vi "Creat Select cmd.vi"(0 "Col":string, 1 "Code":string, 3 "Condtion":string) -> (2 "连接的字符串":string, 4 "Str":string)   [LabVIEW 2014]
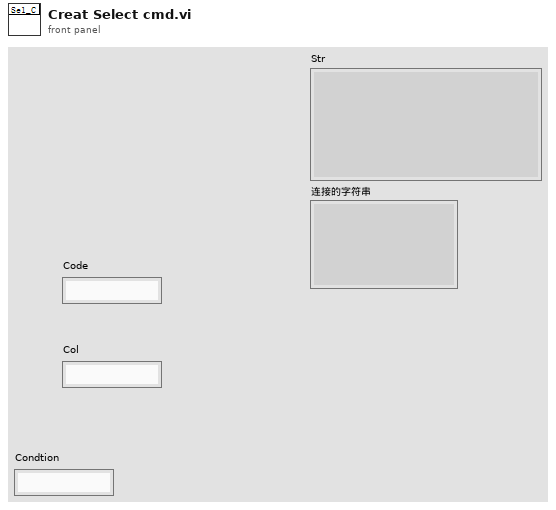
[diagram p1: front panel]
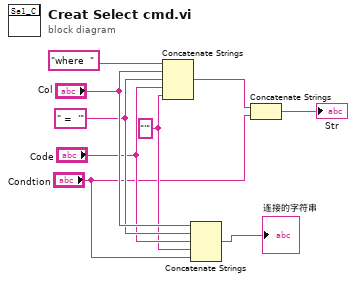
[diagram p0: block diagram]
diagram:
  w2 = "'" ("字符串")
  w5 = " =  '"
  n1 = Concatenate Strings("where  ", "Col", w5, "Code", w2) -> (w8:string)
  n2 = Concatenate Strings("Col", w5, "Code", w2, "Condtion") -> (→"连接的字符串":string)
  n3 = Concatenate Strings(w8, "Condtion") -> (→"Str":string)
